vi "BuildMsg.vi"(5 "Dialog_FPOverwrite?":bool, 7 "BuildType":T1 items=["simple", "Dialog", "PVUpdate", "Dialog&PV", "Asynch", "AsynchDial", "Ack"], 8 "error in (no error)":errorcluster, 9 "ProgressBarCluster":T2, 10 "Msg to be build":string, 11 "CS++Actor in":refnum<class "CS++Actor.lvclass">) -> (0 "error out":errorcluster, 3 "CS++Actor out":refnum<class "CS++Actor.lvclass">)   [LabVIEW 2016, in "CS++Actor.lvlib" / "CS++Actor.lvclass"]
doc: "Build Msg Command."
uses:
  CS++Actor.lvclass
  CSPP_MessageMakerMain/BuildType.ctl
  CSPP_Message/CS++Message.lvclass
  CS++Actor.lvclass/CS++Actor.ctl
  CSPP_Message/CS++Message.lvclass/CS++Message.ctl
  CSPP_MessageMakerMain/CS++MessageMakerMain.lvclass
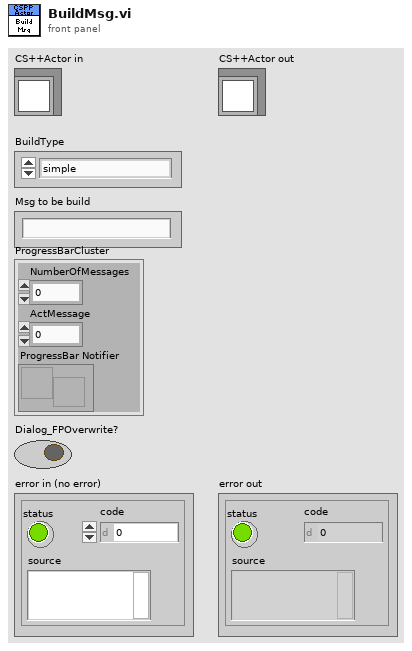
[diagram p1: front panel]
types:
  T1 = typedef "CS++MessageMakerMain.lvlib/CS++MessageMakerMain.lvclass/BuildType.ctl" = u16
  T2 = cluster{"NumberOfMessages":u16, "ActMessage":u16, "ProgressBar Notifier":refnum<notifier>}
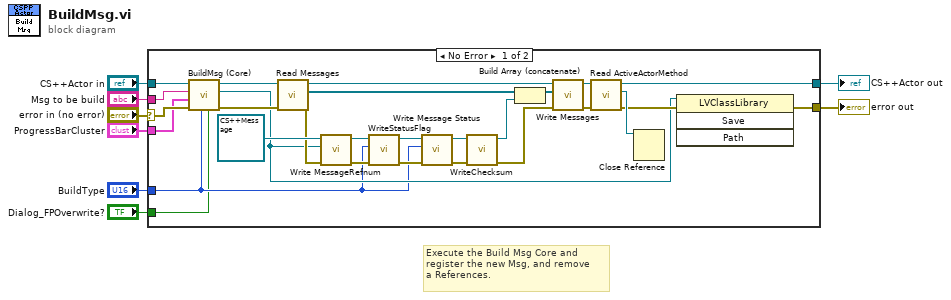
[diagram p0: block diagram]
diagram:
  # "Execute the Build Msg Core and \nregister the new Msg, and remove \na References."
  n1 = case shown="No Error" "error in (no error)" {
    selector: "error in (no error)" -> [w30 w38]
    tunnel: [w20 w38] -> w7
    tunnel: [w22 w37] -> w5
    tunnel: "CS++Actor in" -> [w31 w37]
    tunnel: "Msg to be build" -> [w27 _]
    tunnel: "ProgressBarCluster" -> [w19 _]
    tunnel: "BuildType" -> [w10 _]
    tunnel: "Dialog_FPOverwrite?" -> [w9 _]
    frame No Error {
      n2 = call-dynamic "BuildMsg (Core).vi"("Dialog_FPOverwrite?"=w9, "BuildType"=w10, "error in (no error)"=w30, "ProgressBarCluster"=w19, "Msg to be build"=w27, "CS++Actor in"=w31) -> ("error out"=w29:errorcluster, "ActiveMessageClass"=w21:refnum<vi>, "CS++Actor out"=w28:refnum<class "CS++Actor.lvclass">)  [unwired: 3 in]
      n3 = call "Read Messages.vi"("error in (no error)"=w29, "CS++Actor in"=w28) -> ("error out"=w32:errorcluster, "Messages"=w35:refnum<class "CS++Message.lvclass">[], "CS++Actor out"=w36:refnum<class "CS++Actor.lvclass">)  [unwired: 7 in]
      n4 = call "Write MessageRefnum.vi"("error in (no error)"=w32, "MessageRefnum"=w21, "CS++Message in"=refnum<class "CS++Message.lvclass"> refnum ("CS++Message.lvlib:CS++Message.lvclass")) -> ("error out"=w15:errorcluster, "CS++Message out"=w18:refnum<class "CS++Message.lvclass">)  [unwired: 7 in]
      n5 = call "WriteStatusFlag.vi"("error in (no error)"=w15, "Message Status"=w10, "CS++Message in"=w18) -> ("error out"=w16:errorcluster, "CS++Message out"=w17:refnum<class "CS++Message.lvclass">)  [unwired: 7 in]
      n6 = call "Write Message Status.vi"("error in (no error)"=w16, "Message Status"=w10, "CS++Message in"=w17) -> ("error out"=w12:errorcluster, "CS++Message out"=w14:refnum<class "CS++Message.lvclass">)  [unwired: 7 in]
      n7 = call "WriteChecksum.vi"("error in (no error)"=w12, "CS++Message in"=w14) -> ("error out"=w11:errorcluster, "CS++Message out"=w13:refnum<class "CS++Message.lvclass">)  [unwired: 8 in]
      n8 = Build Array (concatenate)(w35, w13) -> (w34:refnum<class "CS++Message.lvclass">[])
      n9 = call "Write Messages.vi"("error in (no error)"=w11, "Messages"=w34, "CS++Actor in"=w36) -> ("error out"=w25:errorcluster, "CS++Actor out"=w26:refnum<class "CS++Actor.lvclass">)  [unwired: 7 in]
      n10 = call "Read ActiveActorMethod.vi"("error in (no error)"=w25, "CS++Actor in"=w26) -> ("error out"=w23:errorcluster, "ActiveActorMethod"=w24:refnum<vi>, "CS++Actor out"=w22:refnum<class "CS++Actor.lvclass">)  [unwired: 7 in]
      n11 = Close Reference(reference=w24) -> ()  [unwired: 1 in, 1 out]
      n12 = invoke class="LVClassLibrary" method="Save"(reference=w21, error in=w23) -> (error out=w20:errorcluster)  [unwired: 2 in, 3 out]
    }
    frame Error {
    }
  }
  "error out" <- w7
  "CS++Actor out" <- w5
